vi "my old slow dumb vision tracking code.vi"() -> ()   [LabVIEW 2018]
uses:
  <vilib>/vision/NI_Vision_Development_Module.lvlib
panel:
  out "vmax":sgl format="%.2f"
  out "hmin":sgl format="%.2f"
  out "hmax":sgl format="%.2f"
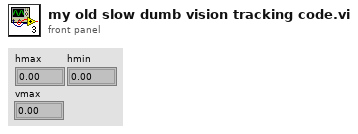
[diagram p1: front panel]
types:
  T1 = cluster{"Left":i32, "Top":i32, "Right":i32, "Bottom":i32, "Bottom 2":i32}
  T2 = typedef "IMAQ Image.ctl" = refnum<image>
  T3 = typedef "IMAQ GM Match Report.ctl" = cluster{"Position":cluster{"x":sgl, "y":sgl}, "Angle":sgl, "Scale":sgl, "Score":sgl, "Bounding Box":cluster{"x":sgl, "y":sgl}[], "Contrast Reversed":bool, "Occlusion %":sgl, "Template Target Curve Score":sgl, "Target Template Curve Score":sgl, "Correlation Score":sgl}
  T4 = cluster{"Calibrated Matches (Pattern Matching 1)[0]":T3, "Calibrated Matches (Pattern Matching 1)[1]":T3, "Calibrated Matches (Pattern Matching 1)[2]":T3, "Calibrated Matches (Pattern Matching 1)[3]":T3, "Calibrated Matches (Pattern Matching 1)[4]":T3, "Calibrated Matches (Pattern Matching 1)[5]":T3, "Calibrated Matches (Pattern Matching 1)[6]":T3, "Calibrated Matches (Pattern Matching 1)[7]":T3, "Calibrated Matches (Pattern Matching 1)[8]":T3}
  T5 = cluster{"Bounding Box[0]":cluster{"x":sgl, "y":sgl}, "Bounding Box[1]":cluster{"x":sgl, "y":sgl}, "Bounding Box[2]":cluster{"x":sgl, "y":sgl}, "Bounding Box[3]":cluster{"x":sgl, "y":sgl}, "Bounding Box[4]":cluster{"x":sgl, "y":sgl}, "Bounding Box[5]":cluster{"x":sgl, "y":sgl}, "Bounding Box[6]":cluster{"x":sgl, "y":sgl}, "Bounding Box[7]":cluster{"x":sgl, "y":sgl}, "Bounding Box[8]":cluster{"x":sgl, "y":sgl}}
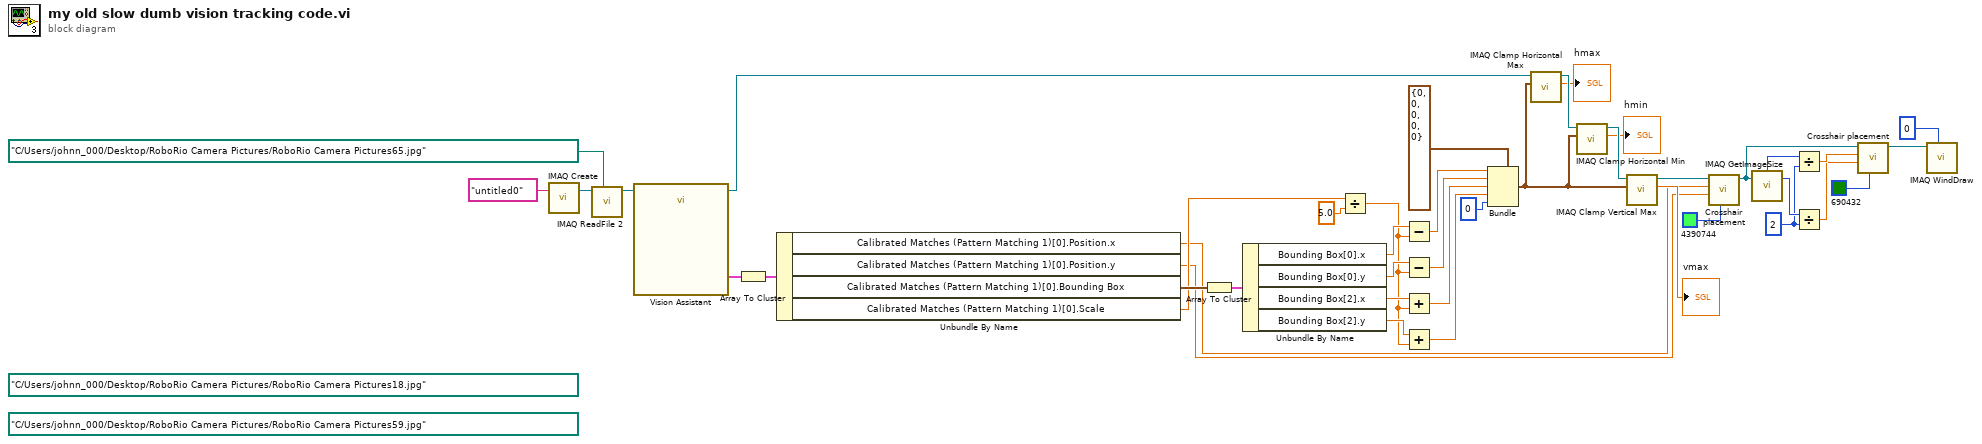
[diagram p0: block diagram]
diagram:
  (unwired) path "C:/Users/johnn_000/Desktop/RoboRio Camera Pictures/RoboRio Camera Pictures18.jpg" ("File Path")
  w6 = 2 ("y")
  (unwired) path "C:/Users/johnn_000/Desktop/RoboRio Camera Pictures/RoboRio Camera Pictures59.jpg" ("File Path")
  n1 = call "IMAQ Create"("Image Name"="untitled0") -> ("New Image"=w41:T2)  [unwired: 4 in, 1 out]
  n2 = call "IMAQ ReadFile 2"("File Path"=path "C:/Users/johnn_000/Desktop/RoboRio Camera Pictures/RoboRio Camera Pictures65.jpg", "Image"=w41) -> ("Image Out"=w14:T2)  [unwired: 5 in, 4 out]
  n3 = call "Vision Assistant"("Image In"=w14) -> ("Image Out"=w31:T2, "Calibrated Matches (Pattern Matching 1)"=w38:T3[])  [unwired: 24 in, 1 out]
  n4 = Array To Cluster(array=w38) -> (cluster=w37:T4)
  n5 = Unbundle By Name(w37) -> ("Calibrated Matches (Pattern Matching 1)[0].Position.x"=w13:sgl, "Calibrated Matches (Pattern Matching 1)[0].Position.y"=w12:sgl, "Calibrated Matches (Pattern Matching 1)[0].Bounding Box"=w36:cluster{"x":sgl, "y":sgl}[], "Calibrated Matches (Pattern Matching 1)[0].Scale"=w17:sgl)
  n6 = Array To Cluster(array=w36) -> (cluster=w35:T5)
  n7 = Unbundle By Name(w35) -> ("Bounding Box[0].x"=w21:sgl, "Bounding Box[0].y"=w20:sgl, "Bounding Box[2].x"=w19:sgl, "Bounding Box[2].y"=w18:sgl)
  n8 = Divide(x=w17, y=sgl 5.0) -> (x/y=w15:sgl)
  n9 = Subtract(x=w21, y=w15) -> (x-y=w25:sgl)
  n10 = Subtract(x=w20, y=w15) -> (x-y=w24:sgl)
  n11 = Add(x=w19, y=w15) -> (x+y=w23:sgl)
  n12 = Add(x=w18, y=w15) -> (x+y=w22:sgl)
  n13 = Bundle(cluster=T1 {"Left"=0, "Top"=0, "Right"=0, "Bottom"=0, "Bottom 2"=0} ("Bounding Rectangle"), "Left"=w25, "Top"=w24, "Right"=w23, "Bottom"=w22, "Bottom 2"=0) -> (w30:T1)
  n14 = call "IMAQ Clamp Horizontal Max"("Rectangle"=w30, "Image"=w31) -> ("Distance"=→"hmax":sgl, "Image Out"=w33:T2)  [unwired: 5 in, 3 out]
  n15 = call "IMAQ Clamp Horizontal Min"("Rectangle"=w30, "Image"=w33) -> ("Distance"=→"hmin":sgl, "Image Out"=w32:T2)  [unwired: 5 in, 3 out]
  n16 = call "IMAQ Clamp Vertical Max"("Rectangle"=w30, "Image"=w32) -> ("Distance"=→"vmax":sgl, "Image Out"=w11:T2)  [unwired: 5 in, 3 out]
  n17 = call "Crosshair placement.vi"("Color"=u32 4390744, "y coordinate"=w12, "x coordinate"=w13, "Image"=w11) -> ("Image Out"=w9:T2)  [unwired: 7 in]
  n18 = call "IMAQ GetImageSize"("Image"=w9) -> ("Y Resolution"=w8:i32, "X Resolution"=w7:i32)  [unwired: 3 in, 1 out]
  n19 = Divide(x=w7, y=w6) -> (x/y=w5:dbl)
  n20 = Divide(x=w8, y=w6) -> (x/y=w4:dbl)
  n21 = call "Crosshair placement.vi"("Color"=u32 690432, "y coordinate"=w4, "x coordinate"=w5, "Image"=w9) -> ("Image Out"=w2:T2)  [unwired: 7 in]
  n22 = call "IMAQ WindDraw"("Window Number (0...15)"=0, "Image"=w2) -> ()  [unwired: 8 in, 2 out]
